vi "HXCPPatten.vi"(11 "stateInfo":T1={"Data storage parameters"={"Name"="", "Format"="TDM", "Connection string"="", "use default"=TRUE}, "Object type"="root", "Selected properties"=[], "Object definitions"=[], "Refnum input wired"=enum."<none>", "Parent object type"="", "Parent object child property"="", "Channel options"=enum."Replace values at index", "PendingCommand"=enum."<none>", "Node style"=enum."Classic", "Only child objects"=FALSE, "TermSpecs"=[], "objectTypeWired"="", "Dynamic format"=FALSE, "Overwrite options"=enum."open or create", "Parameters"=variant, "Format"="", "Node type"=enum."UPDATE", "ImplicitExplicit"=enum."explicit", "Channel type"=enum."Waveform", "Use object with same name"=FALSE, "Show channel terminal"=FALSE, "LabVIEW Version"="", "DataTerminals"=enum."Express", "Size to text"=FALSE, "selected nodes in"=[]}) -> (3 "x .or. y?":bool)   [LabVIEW 2017]
uses:
  <vilib>/Platform/storage/lvStorage.llb/_stateInfoWriteProps.ctl
  <vilib>/Platform/storage/lvStorage.llb/dataStorageParams.ctl
  <vilib>/Platform/storage/lvStorage.llb/_selectedProp.ctl
  <vilib>/Platform/storage/lvStorage.llb/dataModel.ctl
  <vilib>/Platform/storage/Storage.llb/usiTypeDef.ctl
  <vilib>/Platform/storage/Storage.llb/usiPropDef.ctl
  <vilib>/express/express shared/ex_EditUserDefinedProperties/usiDataType.ctl
  <vilib>/Platform/storage/Storage.llb/specialProperties.ctl
  <vilib>/Platform/storage/Storage.llb/usiOverwriteOptions.ctl
  <vilib>/Platform/storage/lvStorage.llb/TerminalDef.ctl
  <vilib>/Platform/storage/lvStorage.llb/_TerminalStyle.ctl
  <vilib>/Utility/XNodeSupport.llb/XRect32.ctl
  <vilib>/Platform/storage/Storage.llb/usiSequenceRepresentation.ctl
  <vilib>/Platform/storage/lvStorage.llb/channelType.ctl
  <vilib>/Platform/storage/lvStorage.llb/_dataTerminals.ctl
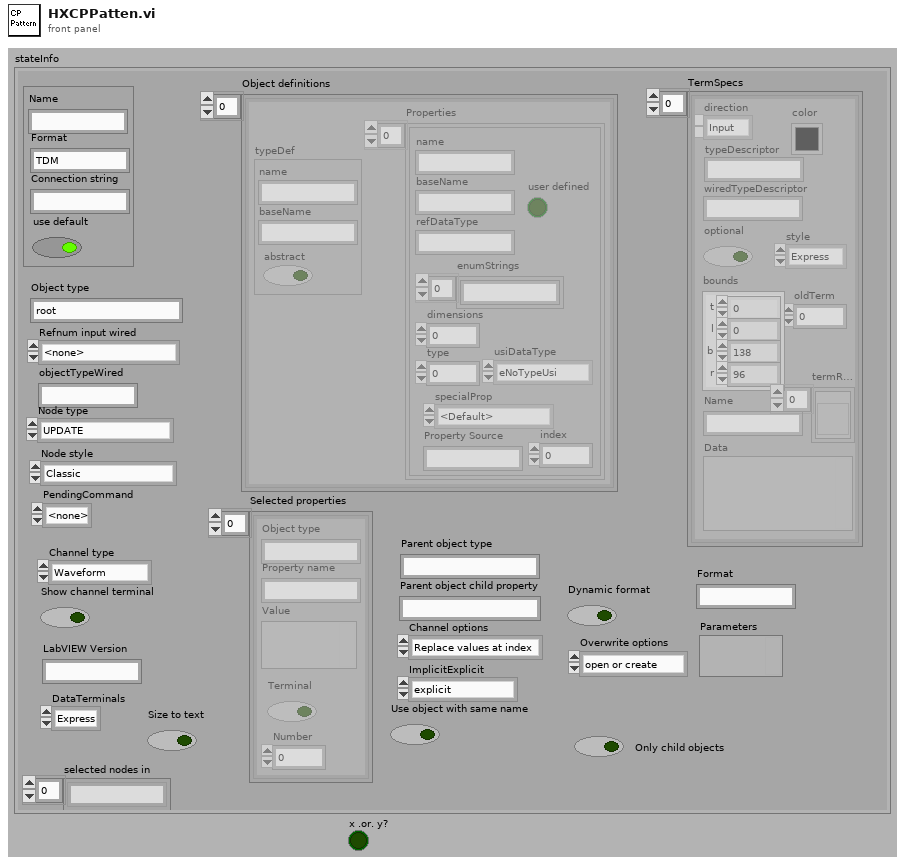
[diagram p1: front panel]
types:
  T1 = typedef "_stateInfoWriteProps.ctl" = cluster{"Data storage parameters":T2, "Object type":string, "Selected properties":T3[], "Object definitions":T4[], "Refnum input wired":enum16{"Storage", "Generic object", "Typed object", "<none>"}, "Parent object type":string, "Parent object child property":string, "Channel options":T9, "PendingCommand":enum16{"<none>", "SelPopUp", "Init"}, "Node style":enum16{"Classic", "Express"}, "Only child objects":bool, "TermSpecs":T10[], "objectTypeWired":string, "Dynamic format":bool, "Overwrite options":enum16{"open", "open or create", "create or replace", "create", "open (read only)"}, "Parameters":variant, "Format":string, "Node type":enum16{"UPDATE", "READ", "QUERY", "CREATE CHILD", "CREATE", "CONNECT", "DISCONNECT"}, "ImplicitExplicit":T13, "Channel type":T14, "Use object with same name":bool, "Show channel terminal":bool, "LabVIEW Version":string, "DataTerminals":T15, "Size to text":bool, "selected nodes in":string[]}
  T2 = typedef "dataStorageParams.ctl" = cluster{"Name":string, "Format":string, "Connection string":string, "use default":bool}
  T3 = typedef "_selectedProp.ctl" = cluster{"Object type":string, "Property name":string, "Value":variant, "Terminal":bool, "Number":i32}
  T4 = typedef "dataModel.ctl" = cluster{"typeDef":T5, "Properties":T6[]}
  T5 = typedef "usiTypeDef.ctl" = cluster{"name":string, "baseName":string, "abstract":bool}
  T6 = typedef "usiPropDef.ctl" = cluster{"name":string, "baseName":string, "refDataType":string, "dimensions":i32, "type":i32, "user defined":bool, "enumStrings":string[], "usiDataType":T7, "specialProp":T8, "Property Source":string, "index":i32}
  T7 = typedef "usiDataType.ctl" = enum16{"eNoTypeUsi", "eInt8Usi", "eInt16Usi", "eInt32Usi", "eInt64Usi", "eUInt8Usi", "eUInt16Usi", "eUInt32Usi", "eUInt64Usi", "eFloat32Usi", "eFloat64Usi", "- 0", "- 1", "- 2", "- 3", "- 4", "- 5", "- 6", "- 7", "- 8", "- 9", "eString8Usi", "eString16Usi", "eStringUsi", "eEnumUsi", "- 10", "- 11", "- 12", "- 13", "- 14", "eTimeUsi", "- 15", "- 16", "- 17", "- 18", "- 19", "- 20", "- 21", "- 22", "- 23", "eInstanceUsi", "eStoreUsi"}
  T8 = typedef "specialProperties.ctl" = enum16{"<Default>", "Channel Values", "AppendReplace", "ChannelFlags", "ValueFlags", "ImplicitExplicit", "InsertIndex", "ValuesCount", "ComparisonOperator", "Cluster", "DAQmx Channel"}
  T9 = typedef "usiOverwriteOptions.ctl" = enum16{"Append values", "Replace values at index", "Replace all values", "Append if timeline aligns"}
  T10 = typedef "TerminalDef.ctl" = cluster{"direction":enum16{"Input", "Output"}, "typeDescriptor":string, "color":u32, "oldTerm":i32, "style":T11, "optional":bool, "bounds":T12, "termRefs":refnum<vi>[], "Name":string, "Data":variant, "wiredTypeDescriptor":string}
  T11 = typedef "_TerminalStyle.ctl" = enum16{"Express", "Collapsed", "Internal"}
  T12 = typedef "XRect32.ctl" = cluster{"t":i32, "l":i32, "b":i32, "r":i32}
  T13 = typedef "usiSequenceRepresentation.ctl" = enum16{"explicit", "implicit"}
  T14 = typedef "channelType.ctl" = enum16{"Waveform", "Array of Double", "Array of String", "DDT", "Array of UInt8", "Array of Int16", "Array of Int32", "Array of Single", "Array of DateTime", "Array of Waveform", "none", "DateTime", "String", "Double", "Single", "UInt8", "Int16", "Int32"}
  T15 = typedef "_dataTerminals.ctl" = enum16{"Express", "Cluster"}
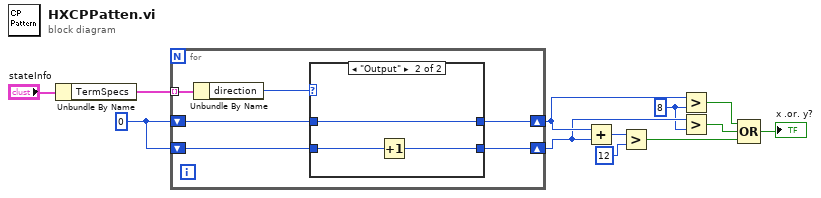
[diagram p0: block diagram]
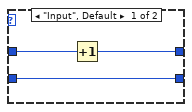
[diagram p2: hidden frame]
diagram:
  w5 = 8 ("y")
  w12 = 0
  n1 = Unbundle By Name("stateInfo") -> ("TermSpecs"=w10:T10[])
  n2 = for {
    tunnel: w10 -> [w18] mode=indexing
    shift-right: [w13] -> w7
    shift-left: w12 -> [w16]
    shift-right: [w14] -> w6
    shift-left: w12 -> [w15]
    n3 = Unbundle By Name(w18) -> ("direction"=w17:enum16{"Input", "Output"})
    n4 = case shown="\"Output\"" w17 {
      tunnel: w16 -> [w20 w24]
      tunnel: w15 -> [w21 w23]
      tunnel: [w21 w22] -> w14
      tunnel: [w19 w24] -> w13
      frame "Input", Default {
        n5 = Increment(x=w20) -> (x+1=w19:i32)
      }
      frame "Output" {
        n6 = Increment(x=w23) -> (x+1=w22:i32)
      }
    }
  }
  n7 = Add(x=w7, y=w6) -> (x+y=w9:i32)
  n8 = Greater?(x=w9, y=12) -> (0:w2:bool)
  n9 = Greater?(x=w7, y=w5) -> (0:w4:bool)
  n10 = Greater?(x=w6, y=w5) -> (0:w3:bool)
  n11 = Compound Arithmetic op=OR(w4, w3, w2) -> (→"x .or. y?":bool)
